vi "Q FGV.vi"(7 "Q Control":T1, 8 "error in (no error)":errorcluster) -> (0 "error out":errorcluster, 3 "queue out":refnum<queue>)   [LabVIEW 2021, in "User Console.lvlib"]
uses:
  User Console.lvlib
  Private Controls/Q Control.ctl
  Private Controls/Q Msg Dataset.ctl
  Private Controls/Module Action.ctl
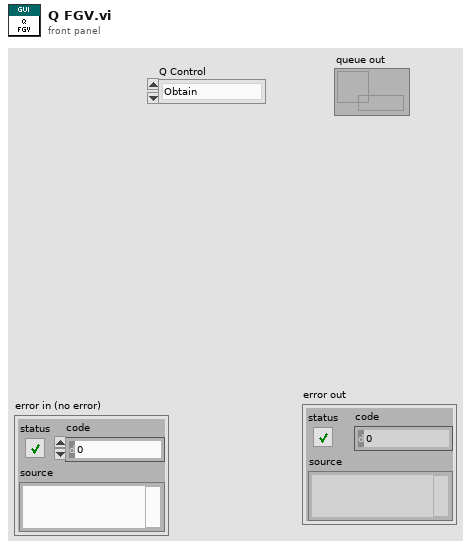
[diagram p1: front panel]
types:
  T1 = typedef "User Console.lvlib/Q Control.ctl" = enum16{"Obtain", "Get", "Release"}
  T2 = typedef "User Console.lvlib/Q Msg Dataset.ctl" = cluster{"Module Action":T3, "Data":variant}
  T3 = typedef "User Console.lvlib/Module Action.ctl" = enum16{"Init", "Error", "Close", "Select Test", "Start Test"}
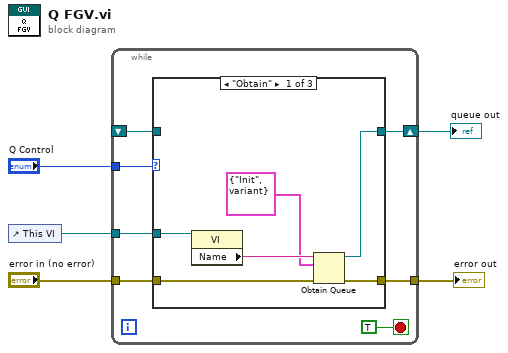
[diagram p0: block diagram]
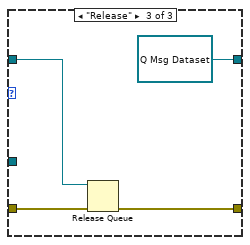
[diagram p3: hidden frame]
diagram:
  n1 = control-ref of="This VI"() -> (w2:refnum<vi>)
  n2 = while {
    tunnel: "Q Control" -> [w11]
    tunnel: "error in (no error)" -> [w10]
    tunnel: [w9] -> w3
    tunnel: w2 -> [w8]
    shift-right: [w7] -> w1
    shift-left: _ -> [w6]
    stop <- TRUE stop-if-true
    n3 = case shown="\"Obtain\"" w11 {
      tunnel: w10 -> [w18 w20 w24]
      tunnel: [w17 w20 w23] -> w9
      tunnel: w8 -> [w16 _ _]
      tunnel: [w13 w19 refnum<queue> refnum ("queue out")] -> w7
      tunnel: w6 -> [_ w19 w22]
      frame "Obtain" {
        n4 = property class="VI"(reference=w16) -> ("Name"=w15:string)  [unwired: 1 in, 2 out]
        n5 = Obtain Queue(name (unnamed)=w15, element data type=T2 {"Module Action"=enum."Init", "Data"=variant} ("Q Msg Dataset"), error in (no error)=w18) -> (queue out=w13:refnum<queue>, error out=w17:errorcluster)  [unwired: 2 in, 1 out]
      }
      frame "Get", Default {
      }
      frame "Release" {
        n6 = Release Queue(queue=w22, error in (no error)=w24) -> (error out=w23:errorcluster)  [unwired: 1 in, 2 out]
      }
    }
  }
  "error out" <- w3
  "queue out" <- w1
